vi "Test_UpstreamError_TransportData_NoWrite_UpstreamErrorReturned.vi"(8 "error in (no error)":errorcluster, 11 "TestCase in":refnum<class "TestITransportAPISemantics.lvclass">) -> (0 "error out":errorcluster, 3 "TestCase out":refnum<class "TestITransportAPISemantics.lvclass">)   [LabVIEW 2017, in "TestITransportAPISemantics.lvclass"]
uses:
  TestITransportAPISemantics.lvclass
  TestITransportAPISemantics.lvclass/TestITransportAPISemantics.ctl
  <vilib>/Utility/error.llb/Error Cluster From Error Code.vi
  <vilib>/ErrorRing/Error Ring.xnode
  Source/ITransport/ITransport.lvclass
panel:
  out "Failed types":string[](array[string])
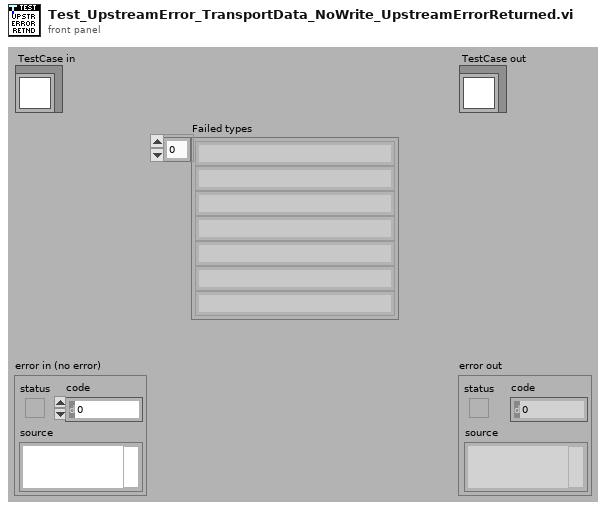
[diagram p1: front panel]
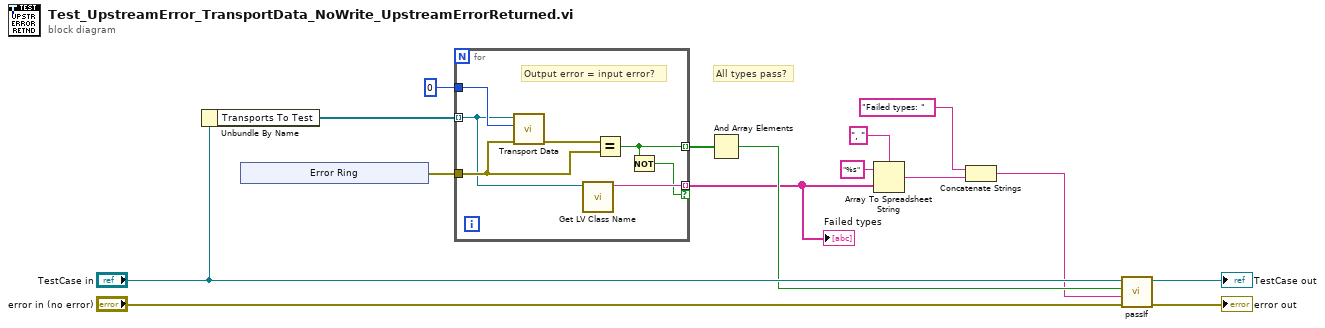
[diagram p0: block diagram]
diagram:
  # "All types pass?"
  n1 = Unbundle By Name("TestCase in") -> ("Transports To Test"=w11:refnum<class "ITransport.lvclass">[])
  n2 = xnode "Error Ring"() -> ("error out"=w10:errorcluster)
  n3 = for {
    tunnel: w11 -> [w19] mode=indexing
    tunnel: w10 -> [w20]
    tunnel: 0 -> [w22]
    tunnel: [w17] -> w8 mode=indexing
    tunnel: [w18] -> w5 mode=indexing if=w16
    # "Output error = input error?"
    n4 = call "Transport Data.vi"("error in (no error)"=w20, "Value"=w22, "ITransport in"=w19) -> ("error out"=w21:errorcluster)  [unwired: 7 in, 1 out]
    n5 = call <vilib>:"Get LV Class Name.vi"("object"=w19) -> ("class name"=w18:string)  [unwired: 9 in, 1 out]
    n6 = Equal?(x=w21, y=w20) -> (x = y?=w17:bool)
    n7 = Not(x=w17) -> (.not. x?=w16:bool)
  }
  "Failed types" <- w5
  n8 = And Array Elements(Boolean array=w8) -> (logical AND=w7:bool)
  n9 = Array To Spreadsheet String(delimiter (Tab)=", ", array=w5, 3:"%s" ("format string")) -> (spreadsheet string=w6:string)
  n10 = Concatenate Strings("Failed types: " ("string"), w6) -> (w2:string)
  n11 = call-dynamic "passIf.vi"("error in (no error)"="error in (no error)", "message (\"\")"=w2, "pass"=w7, "TestCase in"="TestCase in") -> ("error out"=→"error out":errorcluster, "TestCase out"=→"TestCase out":refnum<class "TestITransportAPISemantics.lvclass">)  [unwired: 6 in]
